vi "Update Folder Icon.vi"(0 "TreeControl in":refnum<vi>, 5 "Measurement file Tags":string[](array[string]), 7 "Folder Tag":string, 11 "error in (no error)":errorcluster) -> (4 "TreeControl out":refnum<vi>, 15 "error out":errorcluster)   [LabVIEW 2021, in "Converter.lvlib"]
uses:
  Converter.lvlib
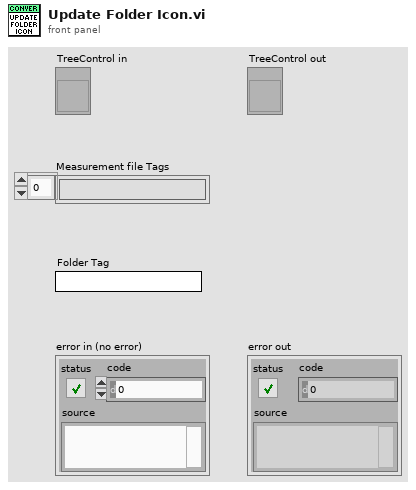
[diagram p1: front panel]
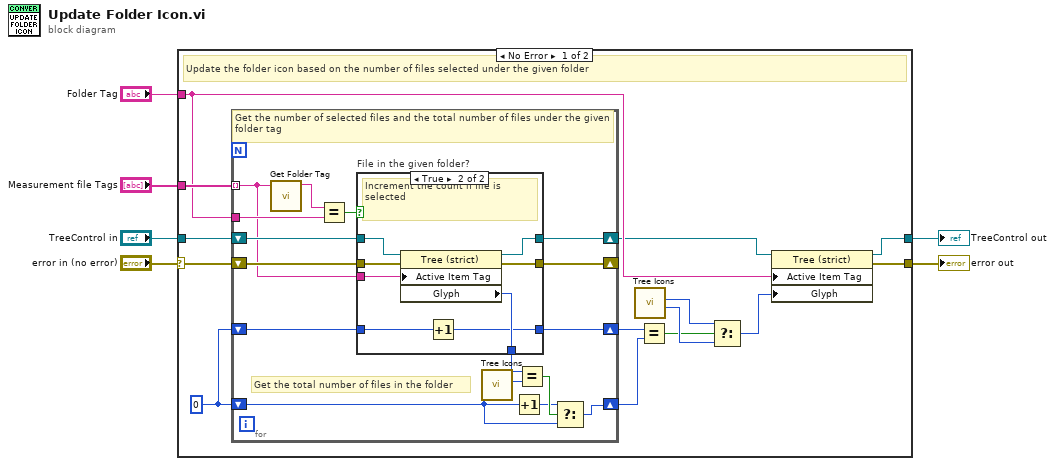
[diagram p0: block diagram]
diagram:
  n1 = case shown="No Error" "error in (no error)" {
    selector: "error in (no error)" -> [w14 w49]
    tunnel: [w16 w49] -> w6
    tunnel: "Folder Tag" -> [w10 _]
    tunnel: "TreeControl in" -> [w13 w48]
    tunnel: "Measurement file Tags" -> [w11 _]
    tunnel: [w12 w48] -> w1
    frame No Error {
      w15 = 0
      # "Update the folder icon based on the number of files selected under the given folder"
      n2 = for {
        tunnel: w10 -> [w36]
        tunnel: w11 -> [w22] mode=indexing
        shift-right: [w33] -> w9
        shift-left: w13 -> [w34]
        shift-right: [w23] -> w7
        shift-left: w15 -> [w29]
        shift-right: [w27] -> _
        shift-left: w14 -> [w26]
        shift-right: [w24] -> w8
        shift-left: w15 -> [w25]
        # "Get the total number of files in the folder"
        # "Get the number of selected files and the total number of files under the given folder tag"
        n3 = call "Get Folder Tag.vi"("Selected cell Tag"=w22) -> ("Folder Tag"=w21:string)  [unwired: 6 in]
        n4 = Equal?(x=w21, y=w36) -> (x = y?=w35:bool)
        n5 = case "File in the given folder?" shown="True" w35 {
          tunnel: w26 -> [w38 w47]
          tunnel: w34 -> [w39 w46]
          tunnel: w22 -> [_ w45]
          tunnel: [w39 w44] -> w33
          tunnel: [w38 w42] -> w27
          tunnel: [_ w43] -> w32
          tunnel: w25 -> [w37 w41]
          tunnel: [w37 w40] -> w24
          frame False {
            # "Pass"
          }
          frame True {
            # "Increment the count if file is selected"
            n6 = property on="Property Node" class="Tree (strict)"(reference=w46, error in=w47, "Active Item Tag"=w45) -> (reference out=w44:refnum<vi>, error out=w42:errorcluster, "Glyph"=w43:i32)
            n7 = Increment(x=w41) -> (x+1=w40:i32)
          }
        }
        n8 = call "Tree Icons.vi"() -> ("Selected"=w28:i32)  [unwired: 6 in, 1 out]
        n9 = Increment(x=w29) -> (x+1=w30:i32)
        n10 = Equal?(x=w32, y=w28) -> (x = y?=w31:bool)
        n11 = Select(t=w30, s=w31, f=w29) -> (s? t:f=w23:i32)
      }
      n12 = call "Tree Icons.vi"() -> ("Not Selected"=w19:i32, "Selected"=w18:i32)  [unwired: 6 in]
      n13 = Equal?(x=w8, y=w7) -> (x = y?=w17:bool)
      n14 = Select(t=w18, s=w17, f=w19) -> (s? t:f=w20:i32)
      n15 = property on="Property Node" class="Tree (strict)"(reference=w9, "Active Item Tag"=w10, "Glyph"=w20) -> (reference out=w12:refnum<vi>, error out=w16:errorcluster)  [unwired: 1 in]
    }
    frame Error {
      # "Pass"
    }
  }
  "TreeControl out" <- w1
  "error out" <- w6
